vi "set_stage (SubVI).vi"(0 "Tot Stage Arr":dbl[](array[numeric]), 1 "Volt vs pos array":cluster{dbl, dbl}[](array[cluster]), 2 "small amp":dbl=1.0 format="%0.2p", 3 "small amp freq":dbl=10.0 format="%0.2p", 4 "Add small amp?":bool, 5 "electrode arr":dbl[][](array[numeric]), 7 "signal type":T1(ring), 9 "electrodes task":refnum<k21>, 11 "electrodes task error":errorcluster, 12 "Num samples":i32, 13 "Use arb force?":bool, 14 "Electrode to sweep":i32) -> (10 "electrodes task 2":refnum<k21>, 15 "electrodes task error 2":errorcluster)   [LabVIEW 2014]
uses:
  <vilib>/DAQmx/write.llb/DAQmx Write (Analog 2D DBL NChan NSamp).vi
  <vilib>/measure/NI_MABase.lvlib
  <resource>/objmgr/daqmx.rc
panel:
  out "Waveform Graph":dbl[][](graph)
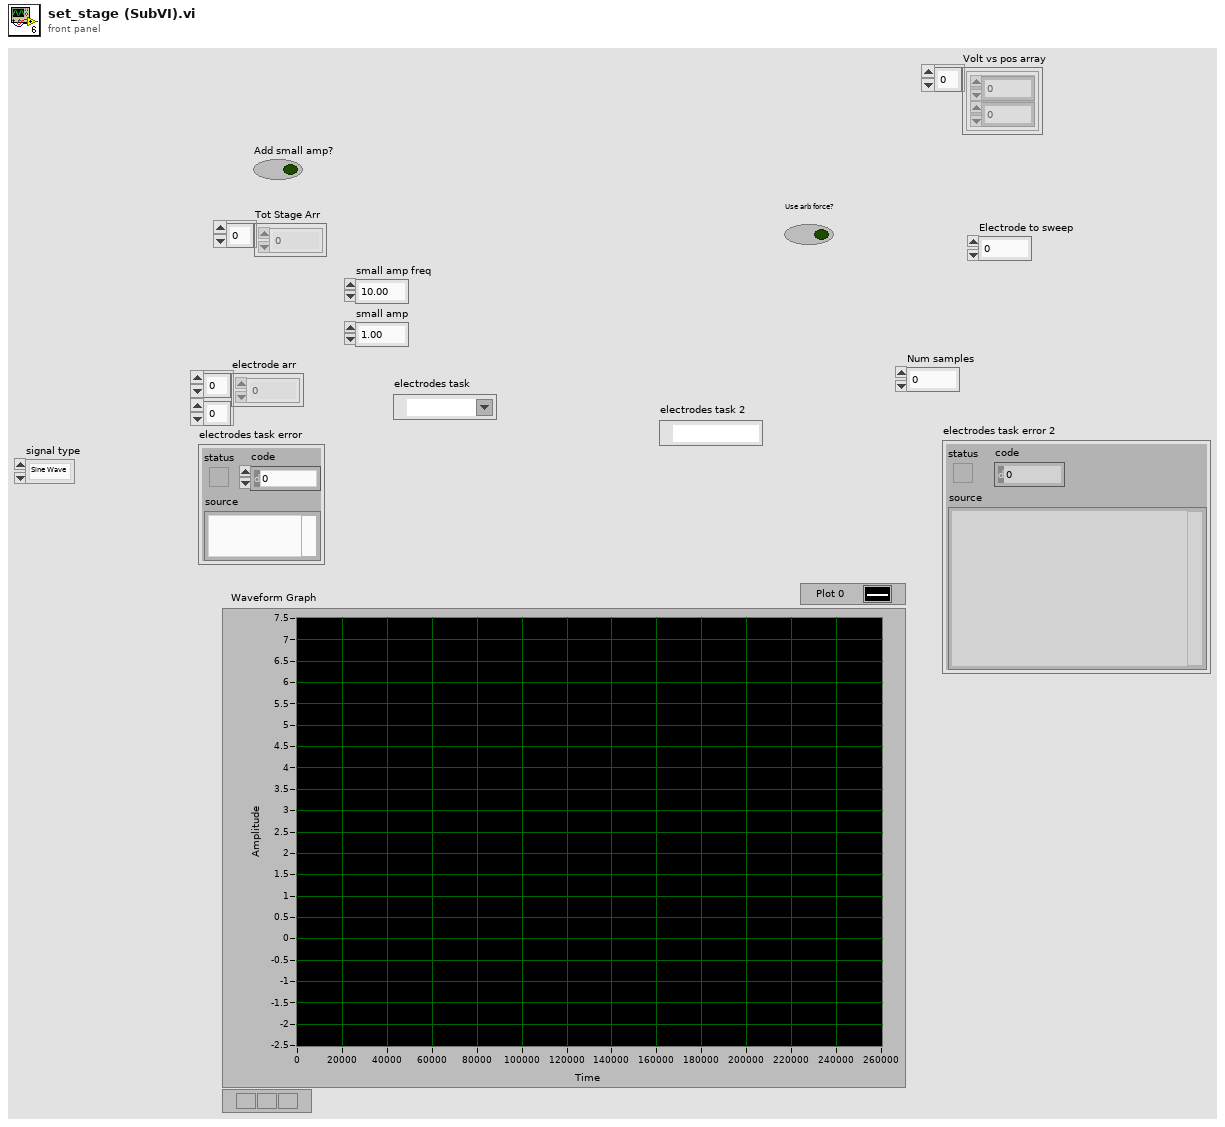
[diagram p1: front panel]
types:
  T1 = enum16{"Sine Wave", "Triangle Wave", "Square Wave", "Sawtooth Wave"}
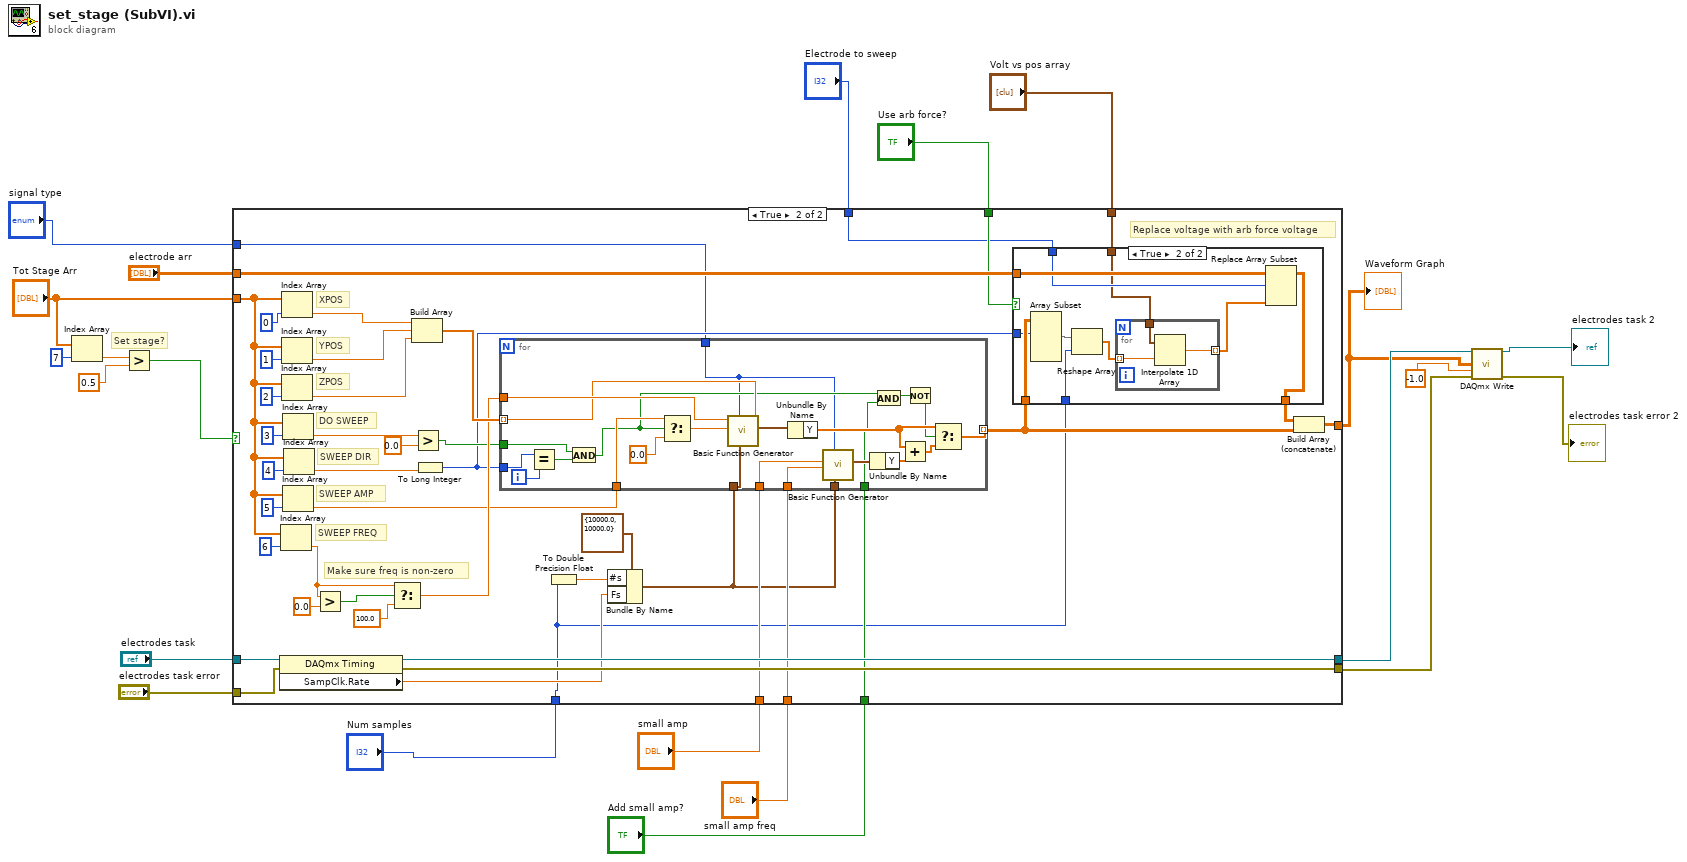
[diagram p0: block diagram]
diagram:
  # "Set stage?"
  n1 = Index Array(array="Tot Stage Arr", index=7) -> (element=w21:dbl)
  n2 = Greater?(x=w21, y=0.5) -> (0:w19:bool)
  n3 = case shown="True" w19 {
    tunnel: "electrode arr" -> [w25 w34]
    tunnel: [w25 w40] -> w9
    tunnel: "Tot Stage Arr" -> [_ w61]
    tunnel: "electrodes task" -> [w24 w56]
    tunnel: "electrodes task error" -> [w23 w55]
    tunnel: [w24 w54] -> w11
    tunnel: [w23 w53] -> w10
    tunnel: "Num samples" -> [_ w27]
    tunnel: "small amp freq" -> [_ w38]
    tunnel: "small amp" -> [_ w37]
    tunnel: "Add small amp?" -> [_ w35]
    tunnel: "Use arb force?" -> [_ w32]
    tunnel: "Electrode to sweep" -> [_ w31]
    tunnel: "Volt vs pos array" -> [_ w28]
    tunnel: "signal type" -> [_ w26]
    frame False {
    }
    frame True {
      # "Replace voltage with arb force voltage"
      # "Make sure freq is non-zero"
      # "SWEEP FREQ"
      # "SWEEP AMP"
      # "SWEEP DIR"
      # "DO SWEEP"
      # "ZPOS"
      # "YPOS"
      # "XPOS"
      n4 = property class="DAQmx Timing"(reference=w56, error in=w55) -> (reference out=w54:refnum<k21>, error out=w53:errorcluster, "SampClk.Rate"=w41:dbl)
      n5 = Index Array(array=w61, index=6) -> (element=w58:dbl)
      n6 = Index Array(array=w61, index=0) -> (element=w51:dbl)
      n7 = Index Array(array=w61, index=1) -> (element=w50:dbl)
      n8 = Index Array(array=w61, index=2) -> (element=w49:dbl)
      n9 = Index Array(array=w61, index=3) -> (element=w46:dbl)
      n10 = Index Array(array=w61, index=5) -> (element=w43:dbl)
      n11 = Index Array(array=w61, index=4) -> (element=w42:dbl)
      n12 = Greater?(x=w58, y=0.0) -> (0:w57:bool)
      n13 = Select(t=w58, s=w57, f=100.0) -> (s? t:f=w47:dbl)
      n14 = Build Array(w51, w50, w49) -> (w48:dbl[])
      n15 = Greater?(x=w46, y=0.0) -> (0:w44:bool)
      n16 = To Long Integer(number=w42) -> (32bit integer=w29:i32)
      n17 = To Double Precision Float(number=w27) -> (double precision float=w39:dbl)
      n18 = Bundle By Name(cluster=cluster{"Fs":dbl, "#s":dbl} {"Fs"=10000.0, "#s"=10000.0} ("sampling info"), "#s"=w39, "Fs"=w41) -> (w36:cluster{"Fs":dbl, "#s":dbl})
      n19 = for {
        tunnel: w48 -> [w105] mode=indexing
        tunnel: w47 -> [w106]
        tunnel: w29 -> [w101]
        tunnel: w36 -> [w100]
        tunnel: [w90] -> w30 mode=indexing
        tunnel: w44 -> [w97]
        tunnel: w43 -> [w96]
        tunnel: w38 -> [w93]
        tunnel: w37 -> [w92]
        tunnel: w36 -> [w91]
        tunnel: w35 -> [w86]
        tunnel: w26 -> [w83]
        i -> [w102]
        n20 = Equal?(x=w101, y=w102) -> (x = y?=w98:bool)
        n21 = And(x=w97, y=w98) -> (x .and. y?=w87:bool)
        n22 = Select(t=w96, s=w87, f=0.0) -> (s? t:f=w104:dbl)
        n23 = call <vilib>:"Basic Function Generator.vi"("offset"=w105, "sampling info"=w100, "signal type"=w83, "amplitude"=w104, "frequency"=w106) -> ("signal out"=w99:waveform(dbl))  [unwired: 4 in, 2 out]
        n24 = Unbundle By Name(w99) -> ("Y"=w88:dbl[])
        n25 = call <vilib>:"Basic Function Generator.vi"("sampling info"=w91, "signal type"=w83, "amplitude"=w92, "frequency"=w93) -> ("signal out"=w95:waveform(dbl))  [unwired: 5 in, 2 out]
        n26 = Unbundle By Name(w95) -> ("Y"=w94:dbl[])
        n27 = And(x=w87, y=w86) -> (x .and. y?=w84:bool)
        n28 = Add(x=w88, y=w94) -> (x+y=w89:dbl[])
        n29 = Not(x=w84) -> (.not. x?=w85:bool)
        n30 = Select(t=w88, s=w85, f=w89) -> (s? t:f=w90:dbl[])
      }
      n31 = case shown="True" w32 {
        tunnel: w34 -> [w69 w79]
        tunnel: [w69 w78] -> w33
        tunnel: w31 -> [_ w77]
        tunnel: w30 -> [_ w76]
        tunnel: w29 -> [_ w75]
        tunnel: w28 -> [_ w71]
        tunnel: w27 -> [_ w70]
        frame False {
        }
        frame True {
          n32 = Array Subset(array=w76, index (row)=w75) -> (w74:dbl[][])  [unwired: 3 in]
          n33 = Reshape Array(w74, w70) -> (w73:dbl[])
          n34 = for {
            tunnel: w73 -> [w82] mode=indexing
            tunnel: [w81] -> w72 mode=indexing
            tunnel: w71 -> [w80]
            n35 = Interpolate 1D Array(1:w82, 2:w80) -> (0:w81:dbl)
          }
          n36 = Replace Array Subset(array=w79, new element=w72, index (row)=w77) -> (w78:dbl[][])  [unwired: 1 in]
        }
      }
      n37 = Build Array (concatenate)(w33, w30) -> (w40:dbl[][])
    }
  }
  "Waveform Graph" <- w9
  n38 = call-poly <vilib>:"DAQmx Write.vi"("task/channels in"=w11, "data"=w9, "timeout"=-1.0, "error in"=w10) -> ("task out"=→"electrodes task 2":refnum<k21>, "error out"=→"electrodes task error 2":errorcluster)  [unwired: 9 in, 1 out]
